vi "Parse SmartCom Message Parameters.vi"(0 "Message":string, 1 "Param Delimiter ([/ ]+)":string="[/ ]+", 3 "'This' name (empty=none)":string, 5 "clear error":errorcluster, 7 "Param Array Contains only from index 3 (F)":bool) -> (13 "Message Subclass":string, 14 "Root Message":string, 15 "Param 1":string, 16 "Param 2":string, 17 "Params":string[](array[string]), 18 "Message Class":string, 19 "Message Exists":bool)   [LabVIEW 2017]
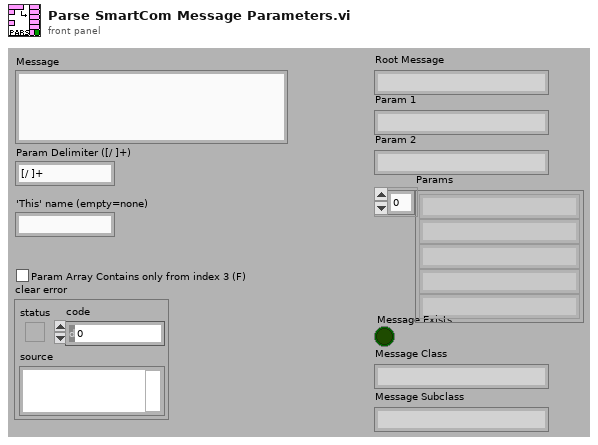
[diagram p1: front panel]
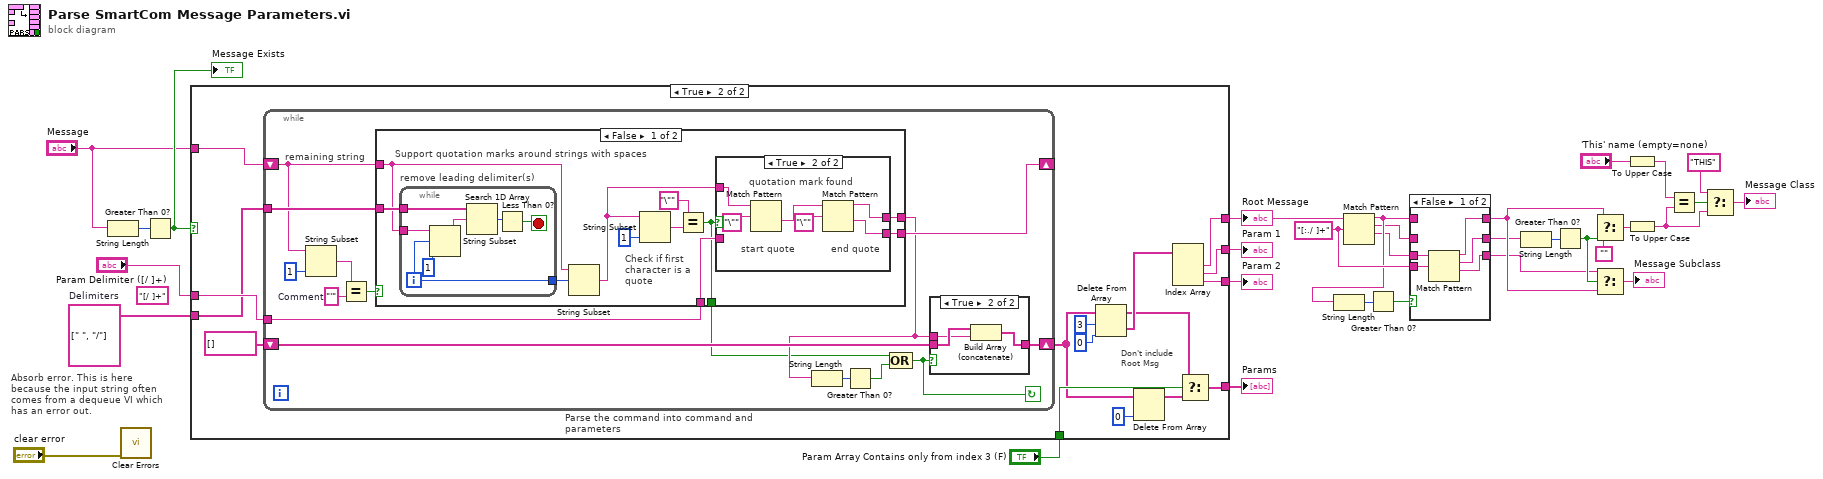
[diagram p0: block diagram]
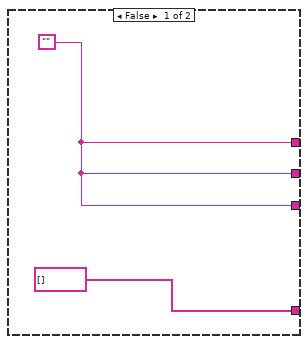
[diagram p3: hidden frame]
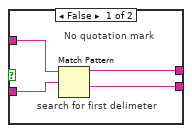
[diagram p4: hidden frame]
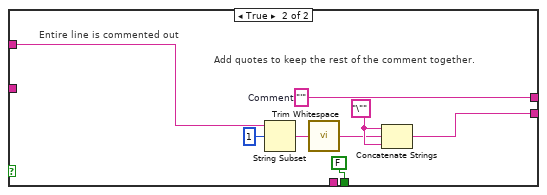
[diagram p5: hidden frame]
diagram:
  w14 = "[:./ ]+" ("regular expression")
  w25 = string[] [" ", "/"]  # Delimiters
  (unwired) "[/ ]+" ("Delimiter [/ ]")
  # "Absorb error. This is here because the input string often comes from a dequeue VI which has an error out."
  n1 = String Length(string="Message") -> (length=w31:i32)
  n2 = call <vilib>:"Clear Errors.vi"("error in (no error)"="clear error") -> ()  [unwired: 5 in, 2 out]
  n3 = Greater Than 0?(x=w31) -> (x > 0?=w30:bool)
  "Message Exists" <- w30
  n4 = case shown="True" w30 {
    tunnel: "Message" -> [_ w47]
    tunnel: "Param Delimiter ([/ ]+)" -> [_ w49]
    tunnel: [w33 w46] -> w21
    tunnel: [w33 w44] -> w29
    tunnel: [w33 w45] -> w28
    tunnel: [string[] [] ("Params") w36] -> w27
    tunnel: w25 -> [_ w42]
    tunnel: "Param Array Contains only from index 3 (F)" -> [_ w39]
    frame False {
      w33 = ""
    }
    frame True {
      # "Don't include Root Msg"
      n5 = while "Parse the command into command and parameters" {
        shift-right: [w61] -> _
        shift-left: w47 -> [w58]
        tunnel: w49 -> [w60]
        shift-right: [w62] -> w35
        shift-left: string[] [] ("Params") -> [w63]
        tunnel: w42 -> [w59]
        stop <- w51 continue-if-true
        w55 = "'"  # Comment
        # "remaining string"
        n6 = String Subset(string=w58, length (rest)=1 ("length (rest)")) -> (substring=w56:string)  [unwired: 1 in]
        n7 = Equal?(x=w56, y=w55) -> (x = y?=w54:bool)
        n8 = case shown="False" w54 {
          tunnel: [w75 w100] -> w53
          tunnel: [w74 w96] -> w61
          tunnel: w60 -> [w73 _]
          tunnel: w59 -> [w71 _]
          tunnel: w58 -> [w66 w99]
          tunnel: [w65 FALSE] -> w50
          frame False {
            # "Support quotation marks around strings with spaces"
            # "Check if first character is a quote"
            n9 = while "remove leading delimiter(s)" {
              tunnel: w71 -> [w81]
              tunnel: [w77] -> w72
              tunnel: w66 -> [w76]
              i -> [w77]
              stop <- w78 stop-if-true
              n10 = String Subset(string=w76, offset (0)=w77, length (rest)=1 ("length (rest)")) -> (substring=w80:string)
              n11 = Search 1D Array(1D array=w81, element=w80) -> (index of element=w79:i32)  [unwired: 1 in]
              n12 = Less Than 0?(x=w79) -> (x < 0?=w78:bool)
            }
            n13 = String Subset(string=w66, offset (0)=w72) -> (substring=w67:string)  [unwired: 1 in]
            n14 = String Subset(string=w67, length (rest)=1 ("length (rest)")) -> (substring=w69:string)  [unwired: 1 in]
            n15 = Equal?(x="\"" ("regular expression"), y=w69) -> (x = y?=w65:bool)
            n16 = case shown="True" w65 {
              tunnel: w67 -> [w86 w90]
              tunnel: w73 -> [w85 _]
              tunnel: [w84 w88] -> w75
              tunnel: [w83 w87] -> w74
              frame False {
                # "search for first delimeter"
                # "No quotation mark"
                n17 = Match Pattern(string=w86, regular expression=w85) -> (before substring=w84:string, after substring=w83:string)  [unwired: 1 in, 2 out]
              }
              frame True {
                # "end quote"
                # "start quote"
                # "quotation mark found"
                n18 = Match Pattern(string=w90, regular expression="\"") -> (after substring=w89:string)  [unwired: 1 in, 3 out]
                n19 = Match Pattern(string=w89, regular expression="\"") -> (before substring=w88:string, after substring=w87:string)  [unwired: 1 in, 2 out]
              }
            }
          }
          frame True {
            w97 = "\""
            w100 = "'"  # Comment
            # "Add quotes to keep the rest of the comment together."
            # "Entire line is commented out"
            n20 = String Subset(string=w99, offset (0)=1) -> (substring=w95:string)  [unwired: 1 in]
            n21 = call <vilib>:"Trim Whitespace.vi"("string"=w95) -> ("trimmed string"=w94:string)  [unwired: 1 in]
            n22 = Concatenate Strings(w97, w94, w97) -> (w96:string)
          }
        }
        n23 = String Length(string=w53) -> (length=w64:i32)
        n24 = Greater Than 0?(x=w64) -> (x > 0?=w52:bool)
        n25 = Compound Arithmetic op=OR(w50, w52) -> (w51:bool)
        n26 = case shown="True" w51 {
          tunnel: w63 -> [w101 w104]
          tunnel: [w101 w102] -> w62
          tunnel: w53 -> [_ w103]
          frame False {
          }
          frame True {
            n27 = Build Array (concatenate)(w104, w103) -> (w102:string[])
          }
        }
      }
      n28 = Delete From Array(array=w35, length=3, index=0) -> (deleted portion=w43:string[], array with subset deleted=w37:string[])
      n29 = Delete From Array(array=w35, index=0) -> (array with subset deleted=w34:string[])  [unwired: 1 in, 1 out]
      n30 = Index Array(array=w43) -> (element #1=w46:string, element #2=w44:string, element #3=w45:string)  [unwired: 3 in]
      n31 = Select(t=w37, s=w39, f=w34) -> (s? t:f=w36:string[])
    }
  }
  "Root Message" <- w21
  "Param 1" <- w29
  "Param 2" <- w28
  "Params" <- w27
  n32 = Match Pattern(string=w21, regular expression=w14) -> (before substring=w13:string, match substring=w11:string, after substring=w9:string)  [unwired: 1 in, 1 out]
  n33 = String Length(string=w13) -> (length=w16:i32)
  n34 = Greater Than 0?(x=w16) -> (x > 0?=w15:bool)
  n35 = case shown="False" w15 {
    tunnel: w14 -> [w109 _]
    tunnel: [w108 w112] -> w12
    tunnel: w13 -> [_ w112]
    tunnel: [w107 w111] -> w10
    tunnel: [w106 w110] -> w8
    tunnel: w11 -> [_ w111]
    tunnel: w9 -> [w105 w110]
    frame False {
      n36 = Match Pattern(string=w105, regular expression=w109) -> (before substring=w108:string, match substring=w107:string, after substring=w106:string)  [unwired: 1 in, 1 out]
    }
    frame True {
    }
  }
  n37 = String Length(string=w10) -> (length=w20:i32)
  n38 = Greater Than 0?(x=w20) -> (x > 0?=w19:bool)
  n39 = Select(t=w12, s=w19, f="") -> (s? t:f=w7:string)
  n40 = Select(t=w8, s=w19, f=w12) -> (s? t:f=→"Message Subclass":string)
  n41 = To Upper Case(1:"'This' name (empty=none)") -> (0:w5:string)
  n42 = To Upper Case(1:w7) -> (0:w3:string)
  n43 = Equal?(x=w5, y=w3) -> (x = y?=w4:bool)
  n44 = Select(t="THIS", s=w4, f=w3) -> (s? t:f=→"Message Class":string)
